vi "Connect To Mb.vi"(0 "reference in":refnum<class "NeedleValve.lvclass">, 5 "modbus":refnum<class "Modbus Master.lvclass">, 11 "error in (no error)":errorcluster) -> (4 "reference out":refnum<class "NeedleValve.lvclass">, 15 "error out":errorcluster)   [LabVIEW 2019, in "NeedleValve.lvclass"]
uses:
  NeedleValve.lvclass
  <vilib>/NI/Modbus Library/API/Master/Modbus Master.lvclass
  NeedleValve.lvclass/NeedleValve.ctl
  modbus engine custom/MB_MODULE_class/MB_MODULE.lvclass/MB_MODULE.ctl
  modbus engine custom/MB_ENGINE_class/Switch Rule and Polarity.ctl
  modbus engine custom/MB_ENGINE_class/cmd enum.ctl
  modbus engine custom/MB_ENGINE_class/MB_ENGINE.lvclass
  D:/GIT H4000/H4000/src/modbus engine custom/MB_MODULE_class/MB_MODULE.lvclass
  modbus engine custom/MB_MODULE_class/MB_MODULE.lvclass
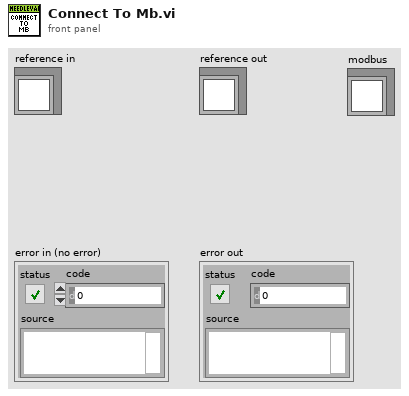
[diagram p1: front panel]
types:
  T1 = typedef "MB_ENGINE.lvclass/Settings.ctl" = cluster{"ACC Steps Per Sec^2":u16, "DEC Steps Per Sec^2":u16, "Min Velosity Step Per Sec":u16, "Max Velosity Step Per Sec":u16, "MicroStep":u16}
  T2 = typedef "MB_ENGINE.lvclass/Switch Rule and Polarity.ctl" = cluster{"Switch Rule":u8, "Polarity, F - NO, T - NC":bool}
  T3 = typedef "MB_ENGINE.lvclass/cmd enum.ctl" = u16
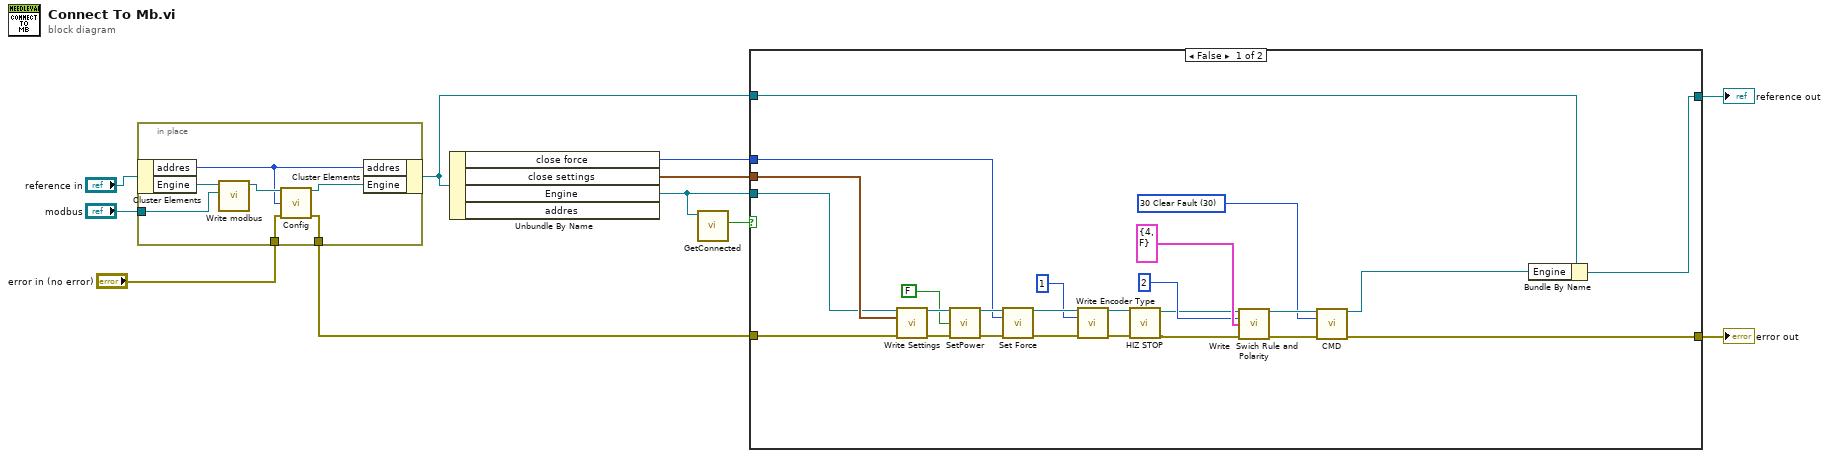
[diagram p0: block diagram]
diagram:
  n1 = in-place {
    in-place-border: "modbus" -> [w18]
    in-place-border: "error in (no error)" -> [w13]
    in-place-border: [w12] -> w1
    n2 = in-place-cluster #1("reference in") -> ("addres"=w14:u16, "Engine"=w17:refnum<class "MB_ENGINE.lvclass">)
    n3 = call "Write modbus.vi"("Modbus Master"=w18, "MB_MODULE in"=w17) -> ("MB_MODULE out"=w16:refnum<class "MB_ENGINE.lvclass">)  [unwired: 9 in]
    n4 = call-dynamic "Config.vi"("class data in"=w16, "addres"=w14, "error in (no error)"=w13) -> ("class data out"=w15:refnum<class "MB_ENGINE.lvclass">, "error out"=w12:errorcluster)  [unwired: 11 in]
    n5 = in-place-cluster #1("addres"=w14, "Engine"=w15) -> (w3:refnum<class "NeedleValve.lvclass">)
  }
  n6 = Unbundle By Name(w3) -> ("close force"=w9:u16, "close settings"=w8:T1, "Engine"=w7:refnum<class "MB_ENGINE.lvclass">)  [unwired: 1 out]
  n7 = call "GetConnected.vi"("MB_MODULE in"=w7) -> ("Connected"=w6:bool)  [unwired: 10 in]
  n8 = case shown="False" w6 {
    tunnel: [w43 w45] -> w11
    tunnel: w1 -> [w20 w44]
    tunnel: w3 -> [w42 w45]
    tunnel: [w41 w44] -> w10
    tunnel: w9 -> [w22 _]
    tunnel: w8 -> [w21 _]
    tunnel: w7 -> [w19 _]
    frame False {
      w24 = T3 30 items=["0 Idle"=0, "1 GoTo Absolute Position"=1, "2 GoTo Relative"=2, "10 GoTo Home Position"=10, "11 Set Home Position"=11, "12 Set FindHome Mode"=12, "13 Reset FindHome Mode"=13, "14 Get FindHome State"=14, "20 Hard Stop"=20, "21 HiZ Stop"=21, "22 Soft Stop"=22, "30 Clear Fault"=30, "40 Encoder Set Home"=40, "70 Driver Init"=70] ("cmd to write")
      n9 = call "Write Settings.vi"("class data in"=w19, "cluster"=w21, "error in (no error)"=w20) -> ("class data out"=w34:refnum<class "MB_ENGINE.lvclass">, "error out"=w39:errorcluster)  [unwired: 11 in]
      n10 = call "SetPower.vi"("class data in"=w34, "On"=FALSE, "error in (no error)"=w39) -> ("class data out"=w35:refnum<class "MB_ENGINE.lvclass">, "error out"=w36:errorcluster)  [unwired: 11 in]
      n11 = call "Set Force.vi"("class data in"=w35, "percent"=w22, "error in (no error)"=w36) -> ("class data out"=w37:refnum<class "MB_ENGINE.lvclass">, "error out"=w38:errorcluster)  [unwired: 11 in]
      n12 = call-dynamic "Write Encoder Type.vi"("class data in"=w37, "U16"=u16 1, "error in (no error)"=w38) -> ("class data out"=w31:refnum<class "MB_ENGINE.lvclass">, "error out"=w30:errorcluster)  [unwired: 11 in]
      n13 = call-dynamic "HIZ STOP.vi"("class data in"=w31, "error in (no error)"=w30) -> ("class data out"=w27:refnum<class "MB_ENGINE.lvclass">, "error out"=w26:errorcluster)  [unwired: 12 in]
      n14 = call-dynamic "Write  Swich Rule and Polarity.vi"("class data in"=w27, "SW"=u16 2, "Switch Rule and Polarity"=T2 {"Switch Rule"=4, "Polarity, F - NO, T - NC"=FALSE}, "error in (no error)"=w26) -> ("class data out"=w25:refnum<class "MB_ENGINE.lvclass">, "error out"=w23:errorcluster)  [unwired: 10 in]
      n15 = call "CMD.vi"("class data in"=w25, "cmd to write"=w24, "error in (no error)"=w23) -> ("class data out"=w40:refnum<class "MB_ENGINE.lvclass">, "error out"=w41:errorcluster)  [unwired: 11 in]
      n16 = Bundle By Name(cluster=w42, "Engine"=w40) -> (w43:refnum<class "NeedleValve.lvclass">)
    }
    frame True {
    }
  }
  "reference out" <- w11
  "error out" <- w10
